vi "RP100ToggleOutput.vi"(2 "error in (no error)":errorcluster, 3 "Enable?":bool, 4 "Source":enum16{"1", "2", "Both"}(ring), 5 "VISA resource name":refnum<visa-resource-name>) -> (0 "error out":errorcluster, 1 "VISA resource name out":refnum<visa-resource-name>)   [LabVIEW 2023]
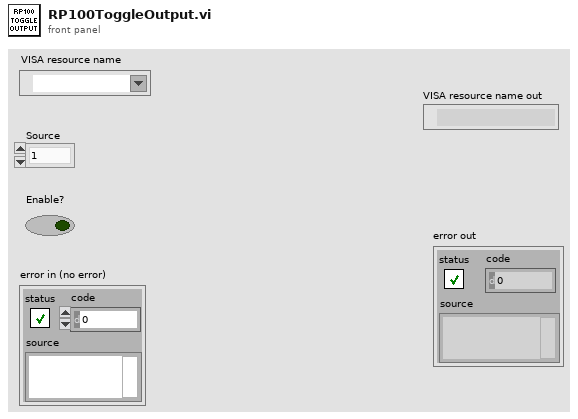
[diagram p1: front panel]
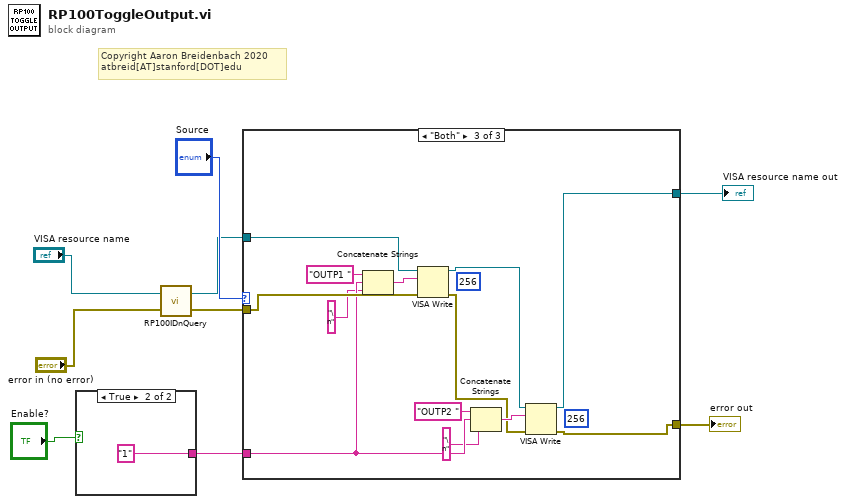
[diagram p0: block diagram]
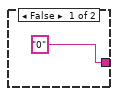
[diagram p2: hidden frame]
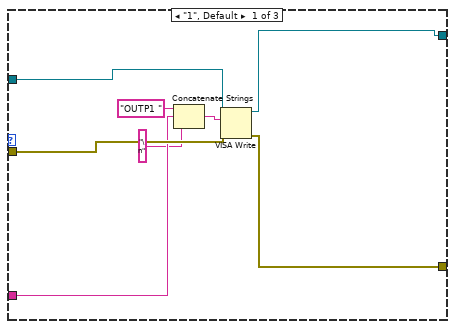
[diagram p3: hidden frame]
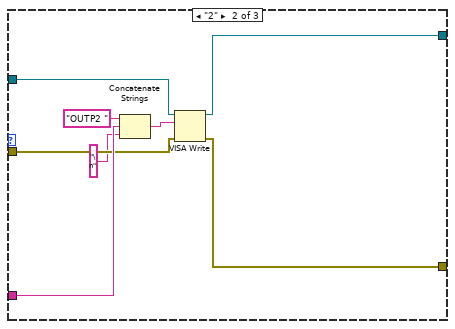
[diagram p4: hidden frame]
diagram:
  # "Copyright Aaron Breidenbach 2020\natbreid[AT]stanford[DOT]edu"
  n1 = case shown="True" "Enable?" {
    tunnel: ["0" "1"] -> w5
    frame False {
    }
    frame True {
    }
  }
  n2 = call "RP100IDnQuery.vi"("error in (no error)"="error in (no error)", "VISA resource name"="VISA resource name") -> ("error out"=w3:errorcluster, "VISA resource name out"=w4:refnum<visa-resource-name>)
  n3 = case shown="\"Both\"" "Source" {
    tunnel: w5 -> [w15 w26 w34]
    tunnel: w4 -> [w17 w24 w37]
    tunnel: w3 -> [w16 w23 w38]
    tunnel: [w12 w20 w29] -> w2
    tunnel: [w13 w21 w28] -> w1
    frame "1", Default {
      n4 = Concatenate Strings("OUTP1 " ("string"), w15, "\n" ("string")) -> (w19:string)
      n5 = VISA Write(VISA resource name=w17, write buffer=w19, error in (no error)=w16) -> (VISA resource name out=w13:refnum<visa-resource-name>, error out=w12:errorcluster)  [unwired: 1 out]
    }
    frame "2" {
      n6 = Concatenate Strings("OUTP2 " ("string"), w26, "\n" ("string")) -> (w27:string)
      n7 = VISA Write(VISA resource name=w24, write buffer=w27, error in (no error)=w23) -> (VISA resource name out=w21:refnum<visa-resource-name>, error out=w20:errorcluster)  [unwired: 1 out]
    }
    frame "Both" {
      (unwired) u32 256 ("byte count")
      (unwired) u32 256 ("byte count")
      n8 = Concatenate Strings("OUTP1 " ("string"), w34, "\n" ("string")) -> (w40:string)
      n9 = VISA Write(VISA resource name=w37, write buffer=w40, error in (no error)=w38) -> (VISA resource name out=w31:refnum<visa-resource-name>, error out=w30:errorcluster)  [unwired: 1 out]
      n10 = Concatenate Strings("OUTP2 " ("string"), w34, "\n" ("string")) -> (w36:string)
      n11 = VISA Write(VISA resource name=w31, write buffer=w36, error in (no error)=w30) -> (VISA resource name out=w28:refnum<visa-resource-name>, error out=w29:errorcluster)  [unwired: 1 out]
    }
  }
  "VISA resource name out" <- w1
  "error out" <- w2
